vi "Recieve Response with Result.vi"(4 "Finished":bool=TRUE, 6 "Result":refnum<class "Mag Lab Result.lvclass">, 8 "error in (no error)":errorcluster, 9 "Requestor":string, 10 "Requestee":string, 11 "Timer test in":refnum<class "Timer test.lvclass">) -> (0 "error out":errorcluster, 3 "Timer test out":refnum<class "Timer test.lvclass">)   [LabVIEW 2015, in "Timer test.lvclass"]
uses:
  Timer test.lvclass
  Mag Lab Result/Mag Lab Result.lvclass
  Mag Lab Result/Timestamp/Timestamp Result.lvclass
  Mag Lab Result/Timestamp/Timestamp Result.lvclass/Timestamp Result.ctl
  Timer test.lvclass/Timer test.ctl
  Mag Lab Root/Mag Lab Root.lvclass/Mag Lab Root.ctl
  <vilib>/ActorFramework/Actor/Actor.lvclass/Actor.ctl
  <vilib>/ActorFramework/Message Enqueuer/Message Enqueuer.lvclass/Message Enqueuer.ctl
  Mag Lab Root Messages/Recieve Request for Result Msg/Recieve Request for Result Msg.lvclass/Recieve Request for Result Msg.ctl
  <vilib>/ActorFramework/Message Enqueuer/Init from Existing Queue.vi
  <vilib>/ActorFramework/Message Enqueuer/Enqueue.vi
  <vilib>/ActorFramework/Message Priority Queue/Priority Enqueue.vi
  <vilib>/ActorFramework/Message Enqueuer/Message Enqueuer.lvclass
  Mag Lab Root Messages/Recieve Request for Result Msg/Recieve Request for Result Msg.lvclass
  <vilib>/ActorFramework/Actor/Actor.lvclass
  Mag Lab Root/Mag Lab Root.lvclass
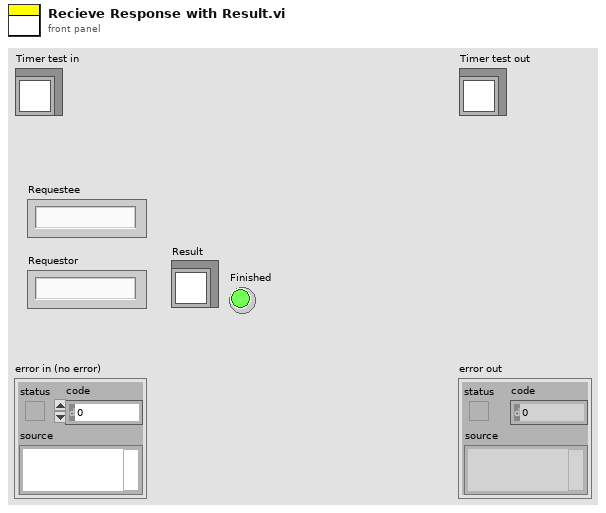
[diagram p1: front panel]
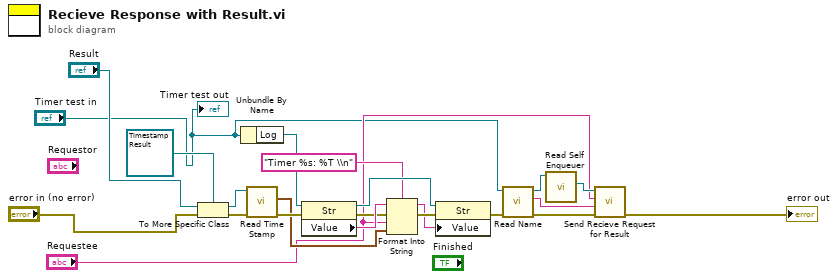
[diagram p0: block diagram]
diagram:
  n1 = To More Specific Class(target class=refnum<class "Timestamp Result.lvclass"> refnum ("Timestamp Result.lvclass"), reference="Result", error in="error in (no error)") -> (specific class reference=w16:refnum<class "Timestamp Result.lvclass">, error out=w15:errorcluster)
  n2 = Unbundle By Name("Timer test in") -> ("Log"=w22:refnum<vi>)
  n3 = call "Read Time Stamp.vi"("error in (no error)"=w15, "Timestamp Result in"=w16) -> ("error out"=w14:errorcluster, "Time Stamp"=w10:timestamp)  [unwired: 7 in, 1 out]
  n4 = property class="Str"(reference=w22, error in=w14) -> (reference out=w21:refnum<vi>, error out=w13:errorcluster, "Value"=w20:string)
  n5 = Format Into String(format string="Timer %s: %T \\n", initial string=w20, error in=w13, "Requestee", w10) -> (resulting string=w11:string, error out=w12:errorcluster)
  n6 = property class="Str"(reference=w21, error in=w12, "Value"=w11) -> (error out=w4:errorcluster)  [unwired: 1 out]
  n7 = call "Read Name.vi"("error in (no error)"=w4, "Mag Lab Root in"="Timer test in") -> ("error out"=w3:errorcluster, "Name"=w5:string, "Mag Lab Root out"=w6:refnum<class "Timer test.lvclass">)  [unwired: 7 in]
  n8 = call <vilib>:"Read Self Enqueuer.vi"("Actor"=w6) -> ("Self Enqueuer"=w8:refnum<class "Message Enqueuer.lvclass">)  [unwired: 10 in]
  n9 = call "Send Recieve Request for Result.vi"("error in (no error)"=w3, "Requestor"=w5, "Requestee"="Requestee", "Message Enqueuer"=w8) -> ("error out"=→"error out":errorcluster)  [unwired: 6 in, 1 out]
  "Timer test out" <- "Timer test in"
